vi "Entorno_Constante(SubVi).vi"(2 "Cluster":cluster{"Translación":dbl[][]}={"Translación"=[[1.0, 1.0, 0.0], [0.0, 0.0, 0.0], [0.0, 0.0, 0.0]]}, 3 "Objetos":path=path "C:/Users/LuisFernando/Documents/UPIITA/8vo semestre/Instrumentacion Virtual Aplicada/Solidworks/Sistema_Coordenado/Archivos Blender/Archivos_constantes") -> (0 "Archivos":i32, 1 "Salida_Texto":string[](array[string]))   [LabVIEW 2017]
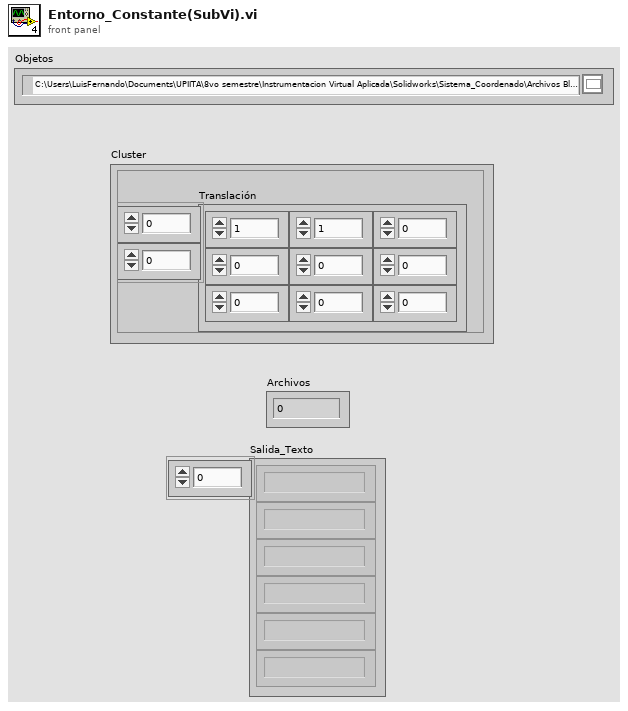
[diagram p1: front panel]
types:
  T1 = cluster{"Escala":dbl[][], "Translación":dbl[][], "Rotación":dbl[][]}
  T2 = enum16{"open", "replace", "create", "open or create", "replace or create", "replace or create with confirmation"}
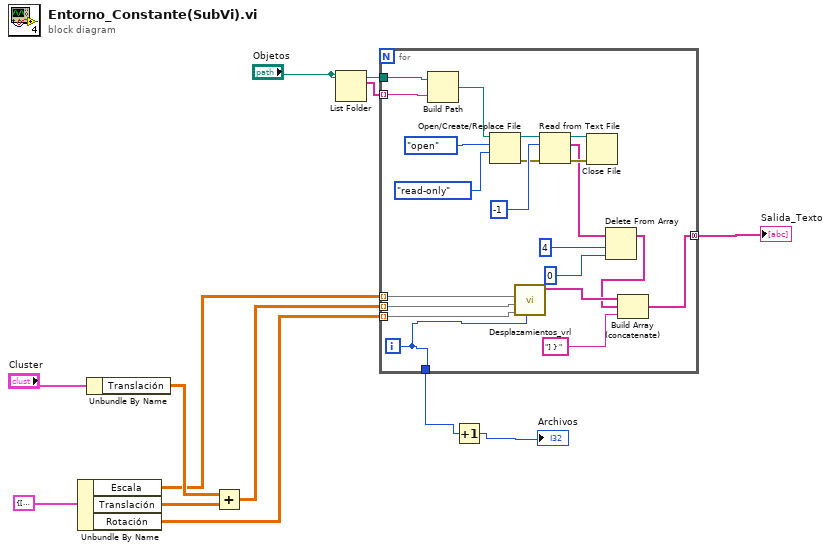
[diagram p0: block diagram]
diagram:
  n1 = Unbundle By Name(T1 {"Escala"=[[0.1, 0.1, 0.1], [1.0, 1.0, 1.0], [1.0, 1.0, 1.0]], "Translación"=[[0.0, -0.75, 0.0], [0.0, 0.0, 0.0], [0.0, 0.0, 0.0]], "Rotación"=[[1.0, 0.0, 0.0, 0.0], [1.0, 0.0, 0.0, 0.0], [1.0, 0.0, 0.0, 0.0]]} ("Cluster_Constante")) -> ("Escala"=w1:dbl[][], "Translación"=w5:dbl[][], "Rotación"=w2:dbl[][])
  n2 = Unbundle By Name("Cluster") -> ("Translación"=w4:dbl[][])
  n3 = Add(x=w4, y=w5) -> (x+y=w3:dbl[][])
  n4 = List Folder(path="Objetos") -> (filenames=w12:string[])  [unwired: 3 in, 3 out]
  n5 = for {
    tunnel: w12 -> [w33] mode=indexing
    tunnel: "Objetos" -> [w32]
    tunnel: [w20] -> w10 mode=concatenating
    tunnel: [w16] -> w8
    tunnel: w3 -> [w15] mode=indexing
    tunnel: w2 -> [w14] mode=indexing
    tunnel: w1 -> [w13] mode=indexing
    i -> [w16]
    n6 = Build Path(base path=w32, name or relative path=w33) -> (appended path=w31:path)
    n7 = Open/Create/Replace File(file path (use dialog)=w31, operation (0:open)=T2."open", access (0:read/write)=enum16{"read/write", "read-only", "write-only"}."read-only") -> (refnum out=w28:refnum<file>, error out=w26:errorcluster)  [unwired: 3 in, 1 out]
    n8 = call "Desplazamientos_vrl.vi"("Indice"=w16, "Rotacion"=w14, "Translacion"=w15, "Escala"=w13) -> ("Salida"=w18:string[])  [unwired: 7 in]
    n9 = Read from Text File(file (use dialog)=w28, count=-1, error in=w26) -> (refnum out=w24:refnum<file>, text=w21:string[], error out=w25:errorcluster)  [unwired: 1 in, 1 out]
    n10 = Close File(refnum=w24, error in=w25) -> ()  [unwired: 2 out]
    n11 = Delete From Array(array=w21, length=4, index=0) -> (array with subset deleted=w17:string[])  [unwired: 1 out]
    n12 = Build Array (concatenate)(w18, w17, "] } ") -> (w20:string[])
  }
  "Salida_Texto" <- w10
  n13 = Increment(x=w8) -> (x+1=→"Archivos":i32)
